vi "Create.vi"(8 "error in (no error)":errorcluster, 10 "Default Namespace":string) -> (0 "error out":errorcluster, 3 "BasicTemplater out":refnum<class "BasicTemplater.lvclass">)   [LabVIEW 2020, in "HTTP Server.lvlib" / "BasicTemplater.lvclass"]
uses:
  BasicTemplater.lvclass
  BasicTemplater.lvclass/BasicTemplater.ctl
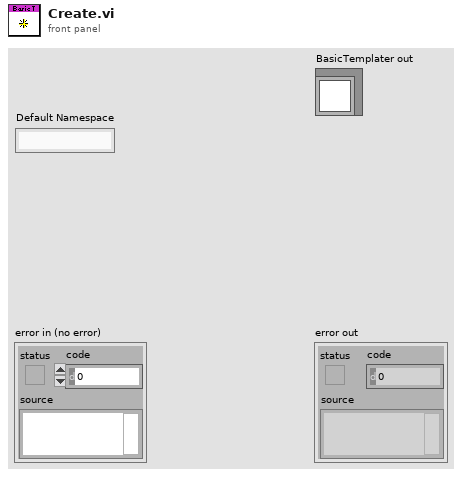
[diagram p1: front panel]
types:
  T1 = map{string, refnum<class "TemplateVariableResolver.lvclass">}
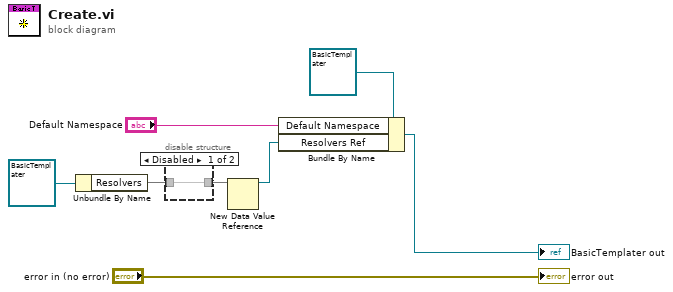
[diagram p0: block diagram]
diagram:
  n1 = Unbundle By Name(refnum<class "BasicTemplater.lvclass"> refnum ("BasicTemplater in")) -> ("Resolvers"=w2:T1)
  n2 = disable-structure shown="Disabled" {
    disable-tunnel: [w9 _] -> w3
    disable-tunnel: w2 -> [w9 _]
    frame Disabled {
    }
    frame Enabled {
    }
  }
  n3 = New Data Value Reference(data value=w3) -> (data value reference=w1:refnum<data-value>)  [unwired: 1 in, 1 out]
  n4 = Bundle By Name(cluster=refnum<class "BasicTemplater.lvclass"> refnum ("BasicTemplater in"), "Default Namespace"="Default Namespace", "Resolvers Ref"=w1) -> (→"BasicTemplater out":refnum<class "BasicTemplater.lvclass">)
  "error out" <- "error in (no error)"
